vi "公式复合写入.vi"(8 "公式":cluster{"X^2":dbl, "X":dbl, "b":dbl}, 9 "量程下拉列表":enum16{"低量程", "高量程"}(ring), 10 "测量模式":T1(ring), 11 "参数下拉列表":u16(ring) items=["总氮"=1, "总磷"=2]) -> ()   [LabVIEW 2016, in "斯坦道总磷.lvlib"]
uses:
  <vilib>/Utility/miscctls.llb/LVPointTypeDef.ctl
panel:
  in  "一键写入":bool
  out "连接的字符串":string
  in  "取消":bool
  in  "确认":bool
  # "请选择要写入的参数"
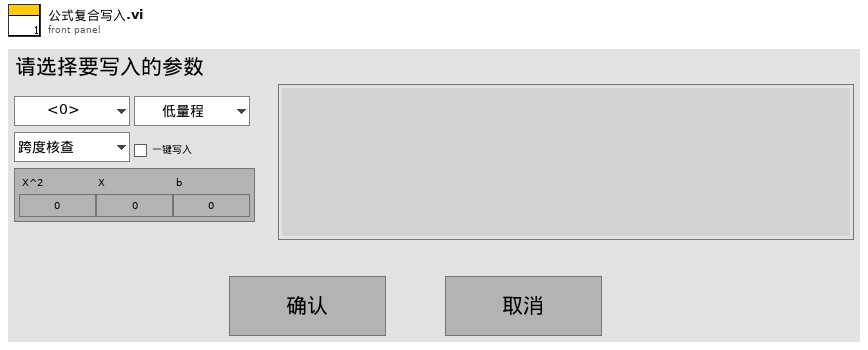
[diagram p1: front panel]
types:
  T1 = enum16{"跨度核查", "水样测量", "零点核查", "标样核查", "加标回收", "快捷测试", "空白校准", "标样校准"}
  T2 = typedef "LVPointTypeDef.ctl" = cluster{"Horizontal":i16, "Vertical":i16}
  T3 = typedef "LVStringsAndValuesArrayTypeDef_U16.ctl" = cluster{"String":string, "Value":u16}[]
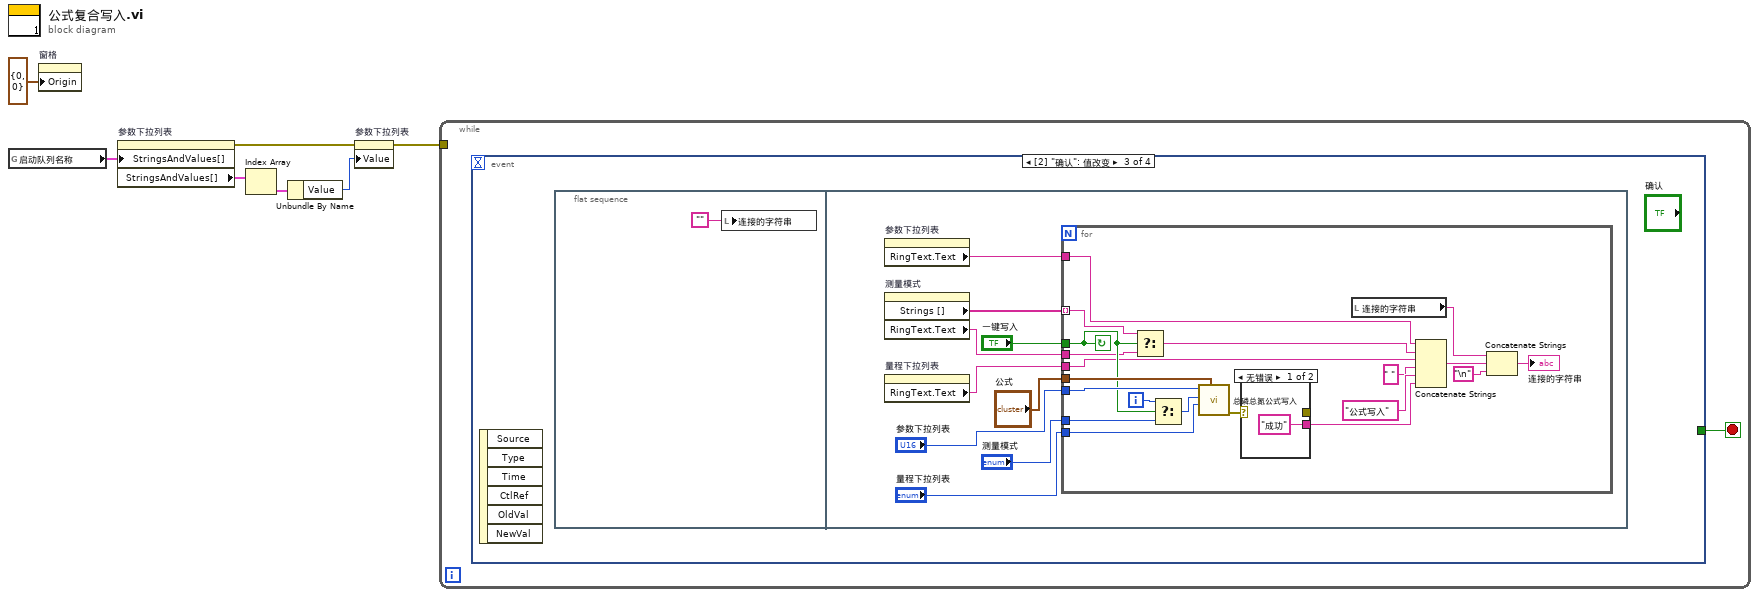
[diagram p0: block diagram]
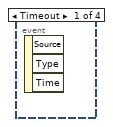
[diagram p2: hidden frame]
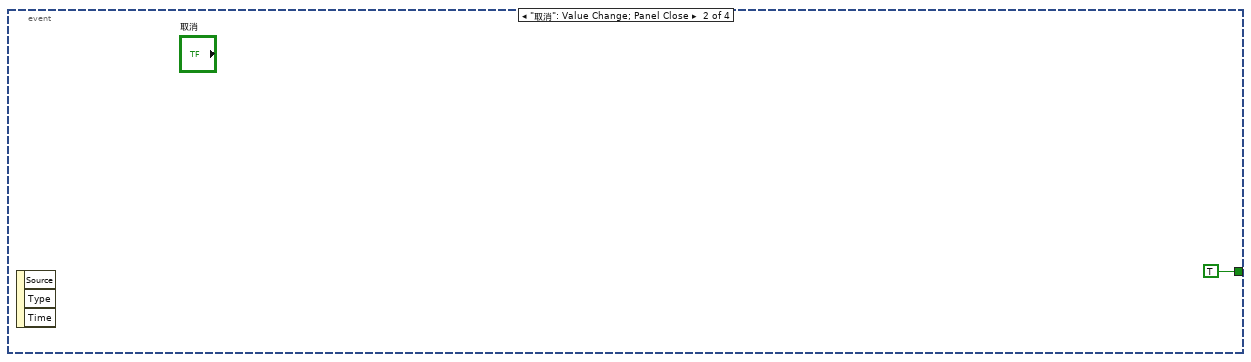
[diagram p3: hidden frame]
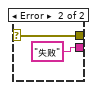
[diagram p4: hidden frame]
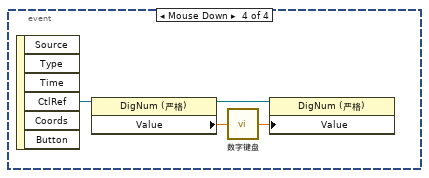
[diagram p5: hidden frame]
diagram:
  n1 = global read "总磷总氮断电保存全局变量.vi" "启动队列名称"() -> (w6:cluster{"String":string, "Value":u16}[])
  n2 = property on="窗格" class="Pane"("Origin"=T2 {"Horizontal"=0, "Vertical"=0} ("原点")) -> ()  [unwired: 2 in, 2 out]
  n3 = property on="参数下拉列表" class="Ring (严格)"("StringsAndValues[]"=w6) -> (error out=w5:errorcluster, "StringsAndValues[]"=w3:T3)  [unwired: 2 in, 1 out]
  n4 = Index Array(array=w3) -> (element=w2:cluster{"String":string, "Value":u16})  [unwired: 1 in]
  n5 = Unbundle By Name(w2) -> ("Value"=w1:u16)
  n6 = property on="参数下拉列表" class="Ring (严格)"(error in=w5, "Value"=w1) -> (error out=w4:errorcluster)  [unwired: 1 in, 1 out]
  n7 = while {
    tunnel: w4 -> [_]
    stop <- w8 stop-if-true
    n8 = event shown="[2] \"确认\": 值改变" {
      selector: _ -> [_ _ _ _]
      dyn-events: _ -> [_ _ _ _]
      timeout: _ -> [_ _ _ _]
      tunnel: [_ TRUE _ _] -> w8
      event Timeout {
        n9 = event-data() -> ()  [unwired: 1 in, 3 out]
      }
      event "取消": Value Change; Panel Close {
        n10 = event-data() -> ()  [unwired: 1 in, 3 out]
      }
      event "确认": Value Change {
        n11 = event-data() -> ()  [unwired: 1 in, 6 out]
        n12 = flat-sequence {
          frame #0 {
            n13 = local write "连接的字符串"("") -> ()
          }
          frame #1 {
            n14 = property on="参数下拉列表" class="Ring (严格)"() -> ("RingText.Text"=w12:string)  [unwired: 2 in, 2 out]
            n15 = property on="测量模式" class="Enum (严格)"() -> ("Strings []"=w16:string[], "RingText.Text"=w15:string)  [unwired: 2 in, 2 out]
            n16 = property on="量程下拉列表" class="Enum (严格)"() -> ("RingText.Text"=w11:string)  [unwired: 2 in, 2 out]
            n17 = for {
              tunnel: "公式" -> [w39]
              tunnel: "参数下拉列表" -> [w35]
              tunnel: "量程下拉列表" -> [w38]
              tunnel: w16 -> [w31] mode=indexing
              tunnel: w15 -> [w30]
              tunnel: "一键写入" -> [w32]
              tunnel: "测量模式" -> [w34]
              tunnel: w12 -> [w22]
              tunnel: w11 -> [w20]
              i -> [w36]
              stop <- w32 continue-if-true
              n18 = Select(t=w31, s=w32, f=w30) -> (s? t:f=w24:string)
              n19 = Select(t=w36, s=w32, f=w34) -> (s? t:f=w33:i32)
              n20 = call "总磷总氮公式写入.vi"("公式"=w39, "量程"=w38, "测量模式"=w33, "测量参数"=w35) -> ("error out"=w37:errorcluster)  [unwired: 7 in]
              n21 = case shown="无错误" w37 {
                selector: w37 -> [_ w42]
                tunnel: [_ w42] -> _
                tunnel: ["成功" "失败"] -> w23
                frame No Error {
                }
                frame Error {
                }
              }
              n22 = local read "连接的字符串"() -> (w25:string)
              n23 = Concatenate Strings(w22, w24, w20, " " ("字符串"), "公式写入", w23) -> (w28:string)
              n24 = Concatenate Strings(w25, w28, "\n") -> (→"连接的字符串":string)
            }
          }
        }
      }
      event "公式.X^2", "公式.X", "公式.b": Mouse Down {
        n25 = event-data() -> ("CtlRef"=w46:refnum<vi>)  [unwired: 1 in, 5 out]
        n26 = property class="DigNum (严格)"(reference=w46) -> (reference out=w43:refnum<vi>, "Value"=w45:dbl)  [unwired: 1 in, 1 out]
        n27 = call "数字键盘.vi"("OldNumber"=w45) -> ("NewNumber"=w44:dbl)
        n28 = property class="DigNum (严格)"(reference=w43, "Value"=w44) -> ()  [unwired: 1 in, 2 out]
      }
    }
  }
